vi "Quick Load Audio File (Core).vi"(8 "error in (no error)":errorcluster, 11 "Path":string) -> (0 "error out":errorcluster, 1 "data":waveform(i16)[](array[waveform]), 2 "Sample Rate":u32, 3 "Channels":u32, 4 "Codec":T1, 5 "PCM Frame Length":u64)   [LabVIEW 2020, in "G-Audio.lvlib"]
doc: "A single VI method to load an entire audio file from disk. The audio data will be returned as an I16 waveform array.\n\nNote this method is faster than reading audio chunks in a loop, but can result in higher peak memory allocation. If the file is very large, LabVIEW may run out of memory.\n\nSupported codecs: flac, mp3, ogg (vorbis), and wav."
uses:
  G-Audio.lvlib
  Controls/Audio File Codec.ctl
  <vilib>/Utility/error.llb/Error Cluster From Error Code.vi
  lib/g_audio_32.dll
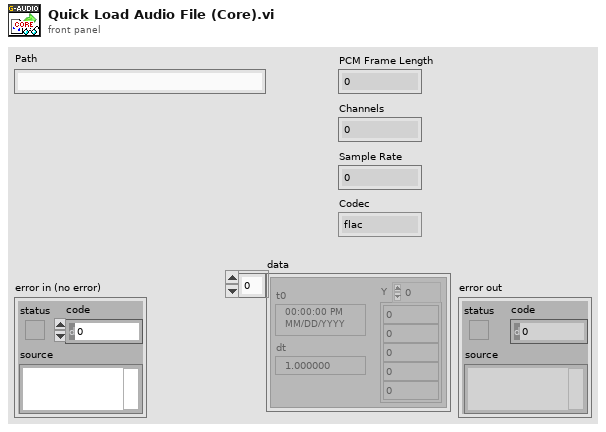
[diagram p1: front panel]
types:
  T1 = typedef "G-Audio.lvlib/Audio File Codec.ctl" = enum16{"flac", "mp3", "vorbis", "wav", "unsupported"}
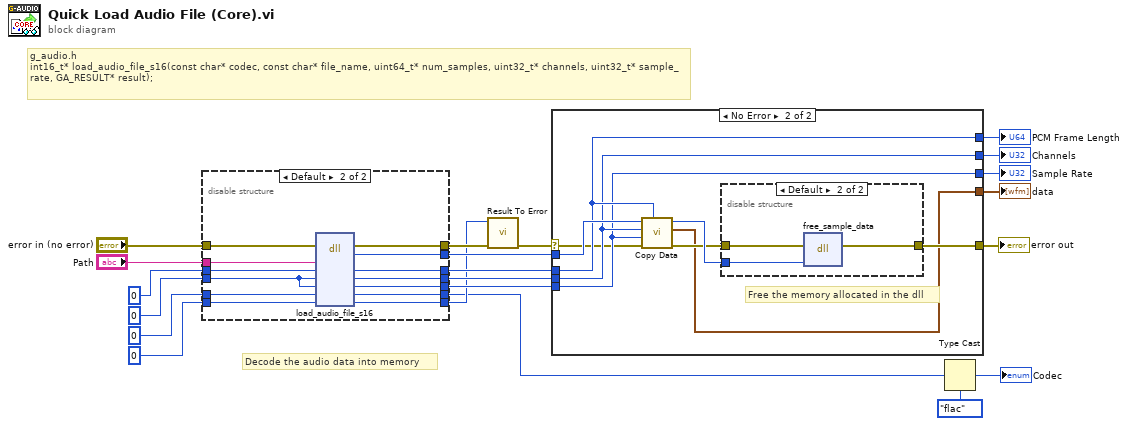
[diagram p0: block diagram]
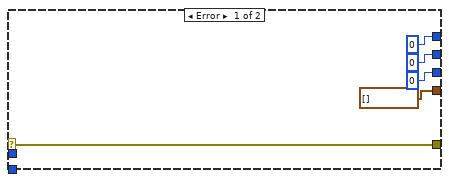
[diagram p2: hidden frame]
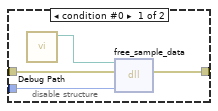
[diagram p3: hidden frame]
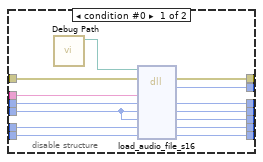
[diagram p4: hidden frame]
diagram:
  # "g_audio.h\nint16_t* load_audio_file_s16(const char* codec, const char* file_name, uint64_t* num_samples, uint32_t* channels, uint32_t* sample_rate, GA_RESULT* result);"
  # "Decode the audio data into memory"
  n1 = disable-structure shown="Default" {
    disable-tunnel: "error in (no error)" -> [w35 w48]
    disable-tunnel: [w33 w46] -> w18
    disable-tunnel: [w32 w45] -> w17
    disable-tunnel: [w31 w44] -> w16
    disable-tunnel: "Path" -> [w29 w42]
    disable-tunnel: [w26 w39] -> w15
    disable-tunnel: [w34 w47] -> w9
    disable-tunnel: u32 0 ("num_samples") -> [w30 w43]
    disable-tunnel: u64 0 ("num_samples") -> [w28 w41]
    disable-tunnel: u16 0 ("num_samples") -> [w24 w37]
    disable-tunnel: [w27 w40] -> w8
    disable-tunnel: 0 ("num_samples") -> [w23 w38]
    disable-tunnel: [w22 w36] -> w5
    frame condition #0 {
      n2 = call "Debug Path.vi"() -> ("Debug Path"=w25:path)  [unwired: 11 in]
      n3 = dll-call lib="?" fn="load_audio_file_s16"(path in=w25, error in=w35, "file_name"=w29, "num_frames"=w28, "channels"=w30, "sample_rate"=w30, "codec"=w24, "result"=w23) -> (error out=w34:errorcluster, "sample_data"=w26:i64, "num_frames"=w33:u64, "channels"=w32:u32, "sample_rate"=w31:u32, "codec"=w22:u16, "result"=w27:i32)  [unwired: 2 in, 1 out]
    }
    frame condition #1 (active) {
      n4 = dll-call lib="C:/github/dataflowg/g-audio/src/LabVIEW/G-Audio/lib/g_audio_*.*" fn="load_audio_file_s16"(error in=w48, "file_name"=w42, "num_frames"=w41, "channels"=w43, "sample_rate"=w43, "codec"=w37, "result"=w38) -> (error out=w47:errorcluster, "sample_data"=w39:i64, "num_frames"=w46:u64, "channels"=w45:u32, "sample_rate"=w44:u32, "codec"=w36:u16, "result"=w40:i32)  [unwired: 3 in, 1 out]
    }
  }
  n5 = call "Result To Error.vi"("error in (no error)"=w9, "Result Code"=w8) -> ("error out"=w7:errorcluster)  [unwired: 9 in]
  n6 = case shown="No Error" w7 {
    selector: w7 -> [w49 w54]
    tunnel: [w49 w62] -> w21
    tunnel: w18 -> [_ w58]
    tunnel: w17 -> [_ w57]
    tunnel: w16 -> [_ w56]
    tunnel: w15 -> [_ w61]
    tunnel: [waveform(i16)[] [] ("Waveform Data") w55] -> w14
    tunnel: [u64 0 ("num_samples") w58] -> w12
    tunnel: [u32 0 ("channels") w57] -> w11
    tunnel: [u32 0 ("sample_rate") w56] -> w10
    frame Error {
    }
    frame No Error {
      # "Free the memory allocated in the dll"
      n7 = call "Copy Data.vi"("num_frames"=w58, "error in (no error)"=w54, "sample_rate"=w56, "channels"=w57, "Data Pointer in"=w61) -> ("error out"=w59:errorcluster, "Waveform Data"=w55:waveform(i16)[], "Data Pointer out"=w60:i64)  [unwired: 4 in]
      n8 = disable-structure shown="Default" {
        disable-tunnel: [w66 w69] -> w62
        disable-tunnel: w60 -> [w65 w68]
        disable-tunnel: w59 -> [w64 w67]
        frame condition #0 {
          n9 = call "Debug Path.vi"() -> ("Debug Path"=w63:path)  [unwired: 11 in]
          n10 = dll-call lib="?" fn="free_sample_data"(path in=w63, error in=w64, "Address (Pointer)"=w65) -> (error out=w66:errorcluster)  [unwired: 3 in, 1 out]
        }
        frame condition #1 (active) {
          n11 = dll-call lib="C:/github/dataflowg/g-audio/src/LabVIEW/G-Audio/lib/g_audio_*.*" fn="free_sample_data"(error in=w67, "Address (Pointer)"=w68) -> (error out=w69:errorcluster)  [unwired: 4 in, 1 out]
        }
      }
    }
  }
  "error out" <- w21
  "PCM Frame Length" <- w12
  "Channels" <- w11
  "Sample Rate" <- w10
  "data" <- w14
  n12 = Type Cast(type=Audio_File_Codec."flac" ("Codec"), x=w5) -> (*(type *) &x=→"Codec":T1)
